vi "Kernel.vi"(0 "ref in":refnum<class "G#RemoteProxy.lvclass">, 1 "object name":string, 2 "option 1":bool, 3 "option 2":bool, 4 "depth":i32, 5 "error in (no error)":errorcluster, 6 "state":T3, 7 "option 3":bool, 8 "attributes in":variant[](array[variant]), 10 "class attributes in":variant[](array[variant])) -> (11 "class attributes out":variant[](array[variant]), 12 "class hierarchy":T1[](array[typedef]), 13 "attributes out":variant[](array[variant]), 14 "ref out":refnum<class "G#RemoteProxy.lvclass">, 15 "AttributeRefs":u32[](array[numeric]), 16 "static attribute ref":u32, 17 "output 1":bool, 18 "output 2":bool, 19 "error out":errorcluster)   [LabVIEW 2017, in "G#RemoteProxy.lvclass"]
doc: "Class kernel, creates and destroys the data value references of the class."
uses:
  G#RemoteProxy.lvclass
  G#Object/utils/G#Object_State.ctl
  G#Object/utils/G#Object_ClassHierarchy.ctl
  protected/ClassAttributesProxy.ctl
  G#Object/G#Object.lvclass
  ClassAttributesRef.ctl
  ObjectAttributesRef.ctl
  protected/ObjectAttributesProxy.ctl
  G#RemoteProxy.lvclass/G#RemoteProxy.ctl
  G#Object/utils/G#Object_ObjectInfoType.ctl
  G#Object/utils/G#Object_CreateMethod.ctl
  G#DebugServer/utils/TCPCommand.ctl
  G#DebugServer/G#DebugServer.lvclass
panel:
  in  "class attributes type":T2
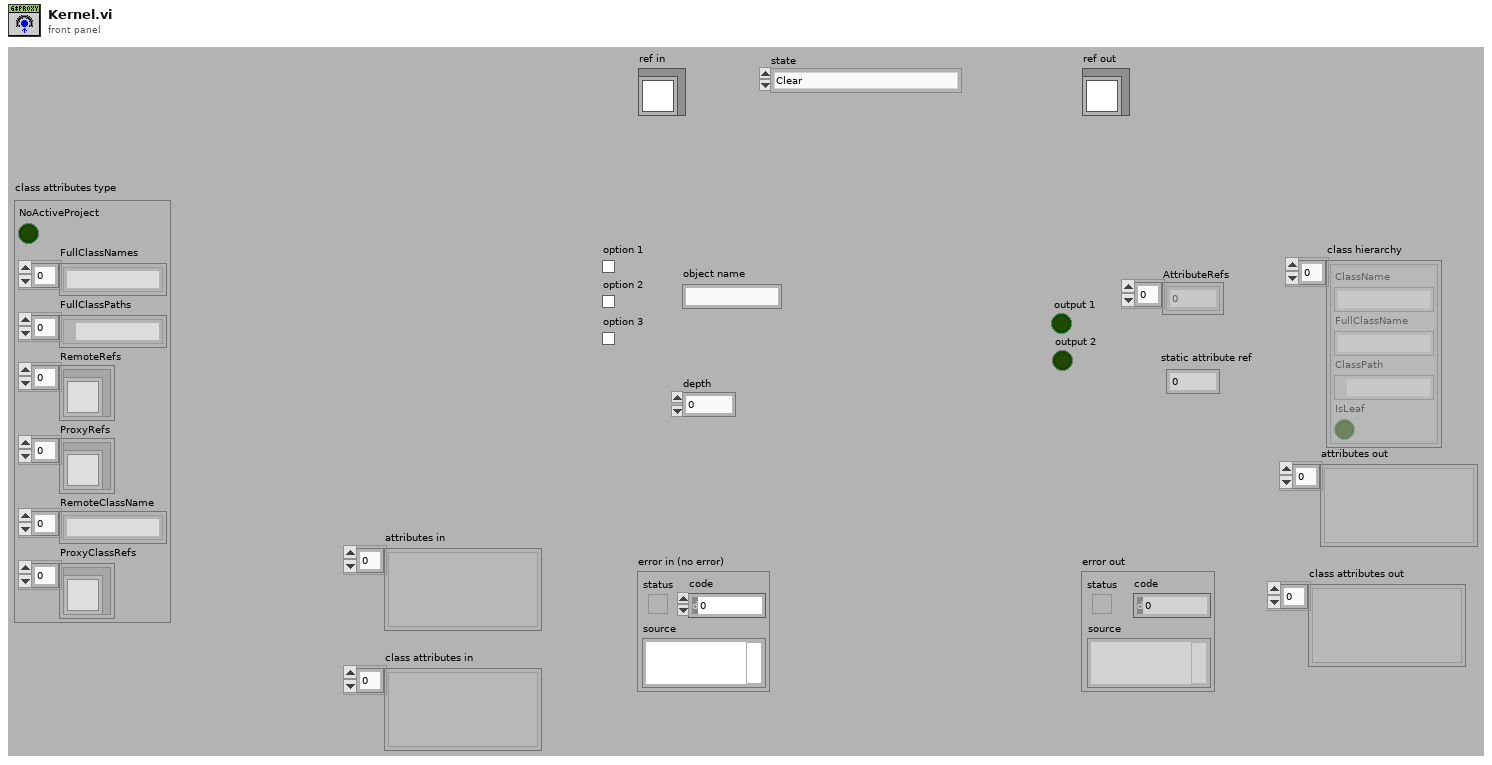
[diagram p1: front panel]
types:
  T1 = typedef "G#Object.lvclass/G#Object_ClassHierarchy.ctl" = cluster{"ClassName":string, "FullClassName":string, "ClassPath":path, "IsLeaf":bool}
  T2 = typedef "G#RemoteProxy.lvclass/ClassAttributesProxy.ctl" = cluster{"NoActiveProject":bool, "FullClassNames":string[], "FullClassPaths":path[], "RemoteRefs":refnum<class "G#Object.lvclass">[], "ProxyRefs":refnum<class "G#RemoteProxy.lvclass">[], "RemoteClassName":string[], "ProxyClassRefs":refnum<class "G#RemoteProxy.lvclass">[]}
  T3 = typedef "G#Object.lvclass/G#Object_State.ctl" = enum16{"Clear", "Create", "Delete", "Get class attributes", "Class hierarchy", "Get attribute value", "Set attribute value"}
  T4 = typedef "G#RemoteProxy.lvclass/ObjectAttributesRef.ctl" = refnum<data-value>
  T5 = typedef "G#RemoteProxy.lvclass/ClassAttributesRef.ctl" = refnum<data-value>
  T6 = typedef "G#RemoteProxy.lvclass/ObjectAttributesProxy.ctl" = cluster{"class hierarchy":T1[], "class name":string, "lvlib hierarchy":string[], "full class name":string, "id":u32, "owner":string, "RemoteRef":refnum<class "G#Object.lvclass">, "object name":string, "attributes":variant[], "connection ID":refnum<k5>, "address":u32, "occurrence":refnum<k4>, "ProxyClassRef":refnum<class "G#RemoteProxy.lvclass">, "InMemory?":bool, "ToString":string}
  T7 = typedef "G#Object.lvclass/G#Object_ObjectInfoType.ctl" = cluster{"ObjectName":string, "ObjectID":u32, "Users":i32, "Counter":bool, "AttributeRefs":u32[], "FullClassName":string, "ClassName":string, "CreateMethod":T8, "GenericDestructorExists":bool, "Owner":string}
  T8 = typedef "G#Object.lvclass/G#Object_CreateMethod.ctl" = enum16{"Create", "Create or look up existing", "Look up existing"}
  T9 = typedef "G#DebugServer.lvclass/TCPCommand.ctl" = u8
  T10 = cluster{"InMemory?":bool, "RemoteRef":refnum<class "G#Object.lvclass">}
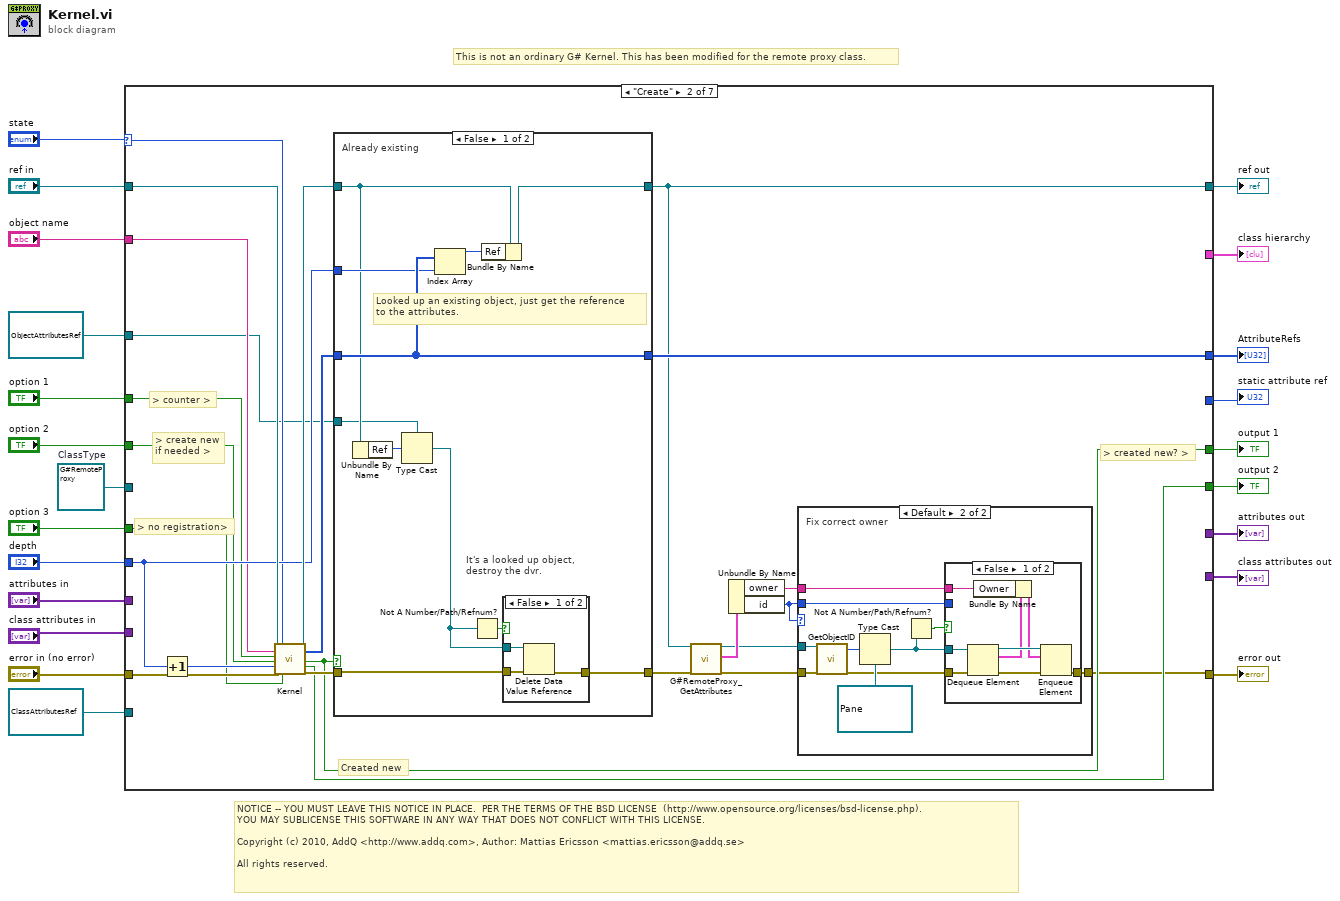
[diagram p0: block diagram]
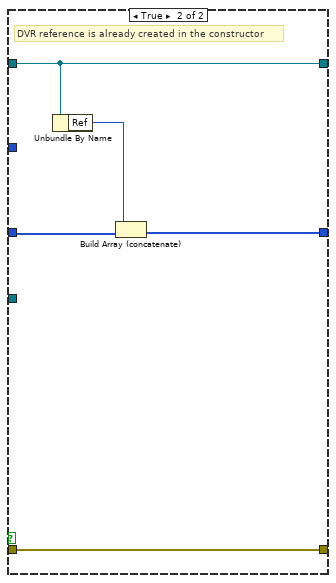
[diagram p6: hidden frame]
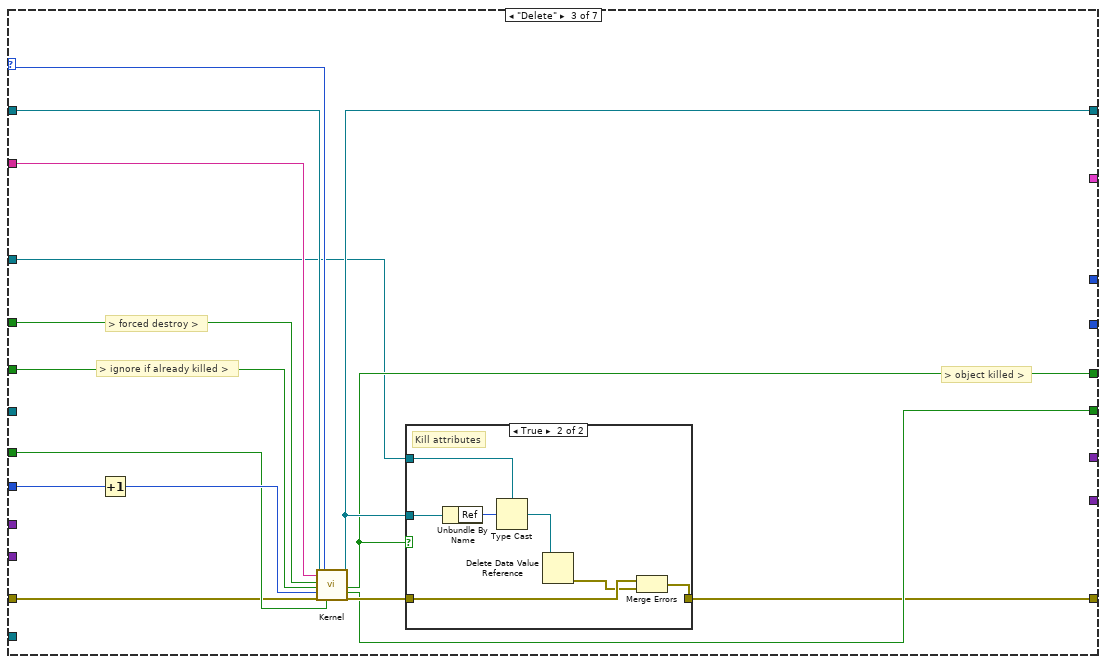
[diagram p7: hidden frame]
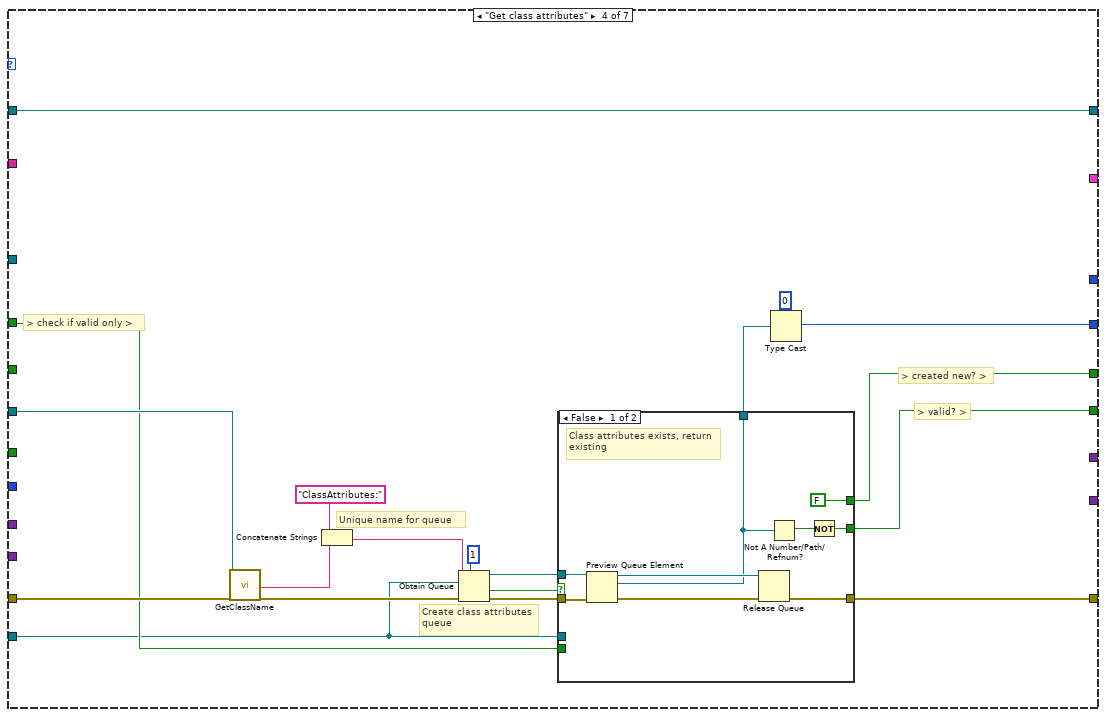
[diagram p9: hidden frame]
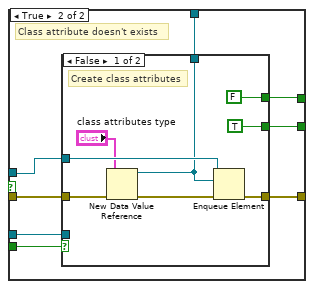
[diagram p10: hidden frame]
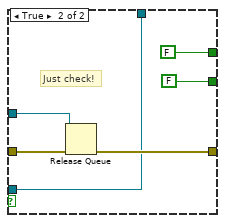
[diagram p11: hidden frame]
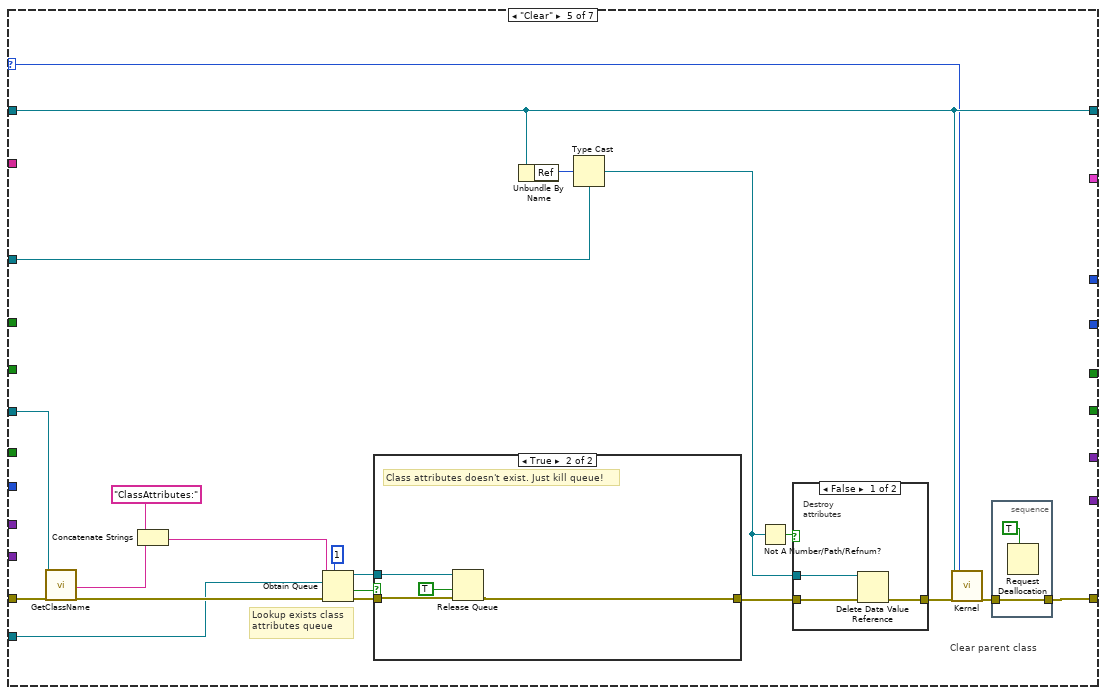
[diagram p12: hidden frame]
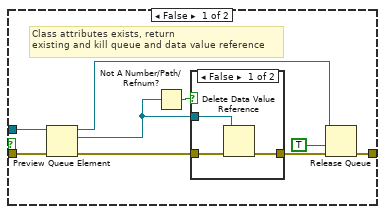
[diagram p14: hidden frame]
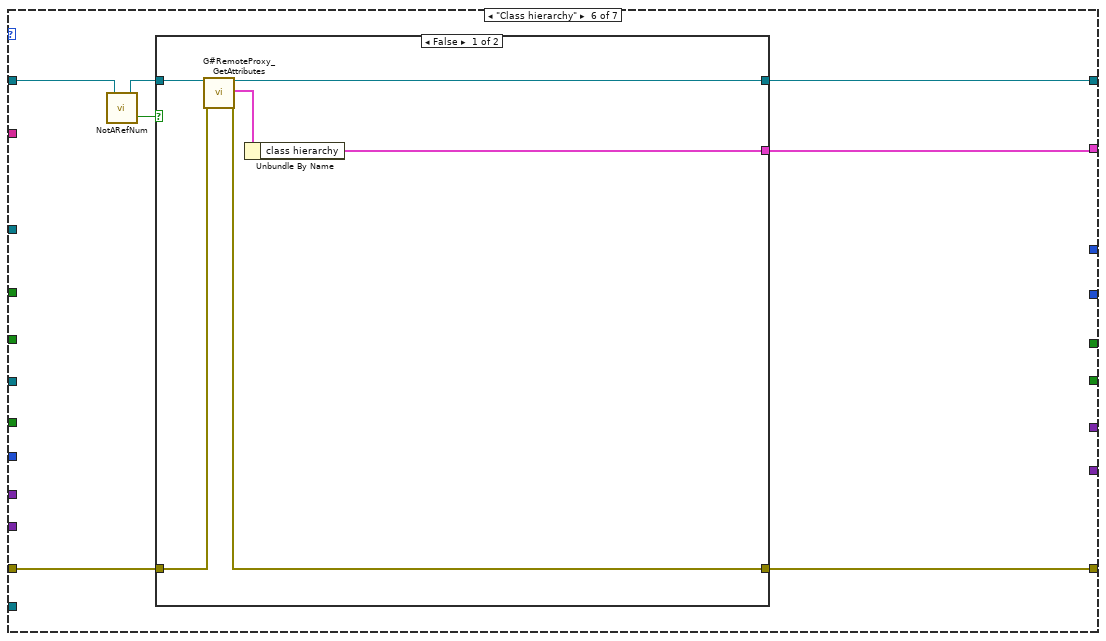
[diagram p16: hidden frame]
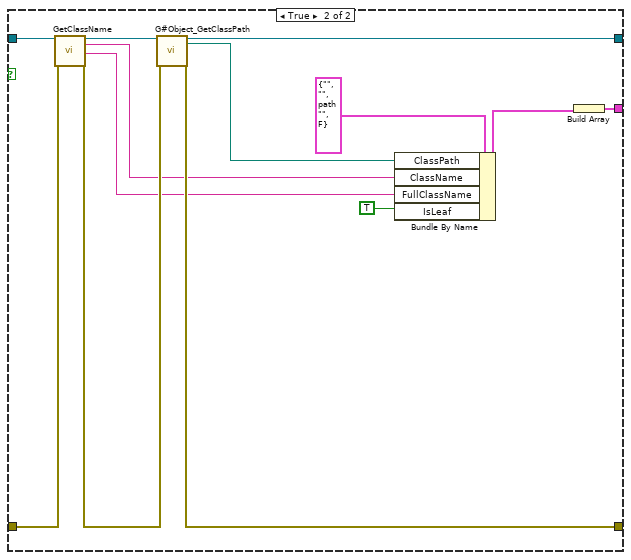
[diagram p17: hidden frame]
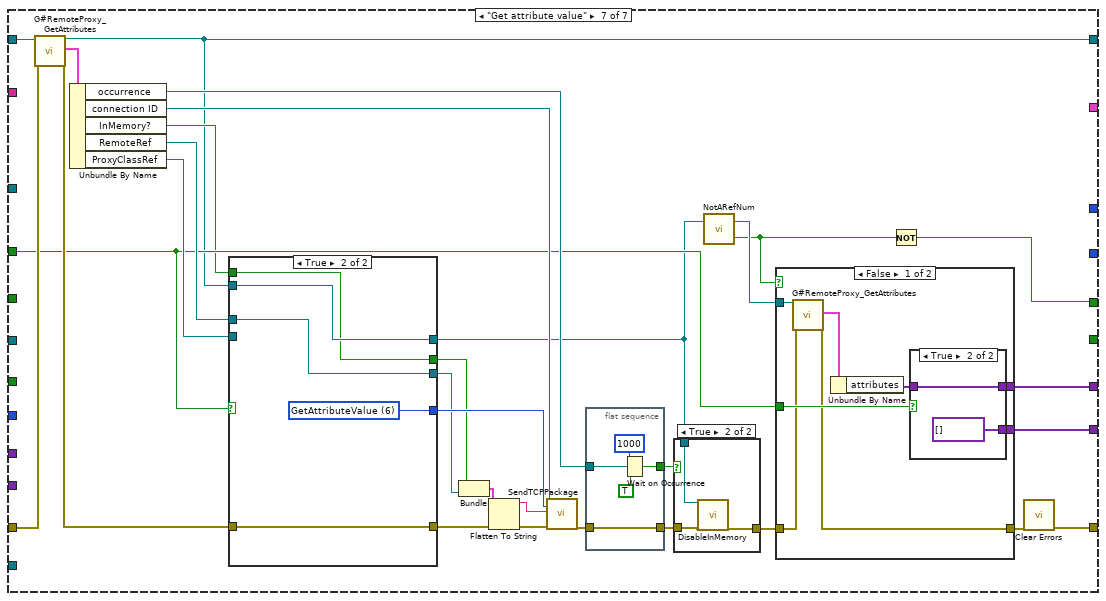
[diagram p18: hidden frame]
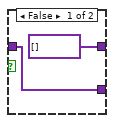
[diagram p19: hidden frame]
diagram:
  w11 = refnum<class "G#RemoteProxy.lvclass"> refnum  # ClassType
  # "This is not an ordinary G# Kernel. This has been modified for the remote proxy class."
  # "NOTICE -- YOU MUST LEAVE THIS NOTICE IN PLACE.  PER THE TERMS OF THE BSD LICENSE  (http://www.opensource.org/licenses/bsd-license.php).\nYOU MAY SUBLICENSE THIS SOFTWARE IN ANY WAY THAT DOES NOT CONFLICT WITH THIS LICENSE.\n\nCopyright (c) 2010, AddQ <http://www.addq.com>, Author: Mattias Ericsson <mattias.ericsson@addq.se>\n\nAll rights reserved."
  n1 = case shown="\"Create\"" "state" {
    selector: "state" -> [_ w41 w99 _ w169 _ _]
    tunnel: "ref in" -> [w24 w45 w96 w130 w170 w208 w261]
    tunnel: [w24 w31 w102 w130 w170 w212 w236] -> w20
    tunnel: "error in (no error)" -> [w23 w44 w91 w129 w182 w211 w260]
    tunnel: [w23 w33 w90 w119 w165 w210 w245] -> w18
    tunnel: "depth" -> [_ w43 w94 _ _ _ _]
    tunnel: "object name" -> [_ w42 w92 _ _ _ _]
    tunnel: "option 1" -> [_ w40 w100 w115 _ _ w246]
    tunnel: [_ w39 _ _ _ _ _] -> w14
    tunnel: [_ w37 w101 w112 _ _ w240] -> w13
    tunnel: [_ _ _ w120 _ _ _] -> w12
    tunnel: w11 -> [_ _ _ w117 w173 _ _]
    tunnel: T5 refnum ("data value reference") -> [_ _ _ w114 w172 _ _]
    tunnel: [_ _ _ _ _ w209 _] -> w9
    tunnel: [_ _ _ _ _ _ w247] -> w8
    tunnel: [_ _ _ _ _ _ w253] -> w7
    tunnel: "option 2" -> [_ w36 w98 _ _ _ _]
    tunnel: "option 3" -> [_ w34 w93 _ _ _ _]
    tunnel: [_ w35 w97 w113 _ _ _] -> w4
    tunnel: "attributes in" -> [_ _ _ _ _ _ _]
    tunnel: "class attributes in" -> [_ _ _ _ _ _ _]
    tunnel: T4 refnum ("attributes ref") -> [_ w25 w89 _ w163 _ _]
    frame Default {
    }
    frame "Create" {
      # "Created new"
      # "> no registration>"
      # "> create new\nif needed >"
      # "> created new? >"
      # "> counter >"
      n2 = Increment(x=w43) -> (x+1=w38:i32)
      n3 = call-parent "Kernel.vi"("reference in"=w45, "object name"=w42, "option 1"=w40, "option 2"=w36, "depth"=w38, "error in (no error)"=w44, "state"=w41, "option 3"=w34) -> ("reference out"=w46:refnum<class "G#RemoteProxy.lvclass">, "attribute refs"=w47:u32[], "output 1"=w37:bool, "output 2"=w35:bool, "error out"=w48:errorcluster)  [unwired: 3 in, 4 out]
      n4 = case shown="False" w37 {
        tunnel: w48 -> [w71 w84]
        tunnel: [w72 w84] -> w32
        tunnel: w46 -> [w75 w86]
        tunnel: [w79 w86] -> w31
        tunnel: w47 -> [w78 w88]
        tunnel: [w78 w87] -> w39
        tunnel: w43 -> [w77 _]
        tunnel: w25 -> [w73 _]
        frame False {
          # "It's a looked up object,\ndestroy the dvr."
          # "Looked up an existing object, just get the reference\nto the attributes."
          # "Already existing"
          n5 = Unbundle By Name(w75) -> ("Ref"=w74:u32)
          n6 = Type Cast(type=w73, x=w74) -> (*(type *) &x=w70:T4)
          n7 = Index Array(array=w78, index=w77) -> (element=w76:u32)
          n8 = Not A Number/Path/Refnum?(number/path/refnum=w70) -> (NaN/Path/Refnum?=w69:bool)
          n9 = Bundle By Name(cluster=w75, "Ref"=w76) -> (w79:refnum<class "G#RemoteProxy.lvclass">)
          n10 = case shown="False" w69 {
            tunnel: [w82 w83] -> w72
            tunnel: w71 -> [w81 w83]
            tunnel: w70 -> [w80 _]
            frame False {
              n11 = Delete Data Value Reference(data value reference=w80, error in=w81) -> (error out=w82:errorcluster)  [unwired: 1 out]
            }
            frame True {
            }
          }
        }
        frame True {
          # "DVR reference is already created in the constructor"
          n12 = Unbundle By Name(w86) -> ("Ref"=w85:u32)
          n13 = Build Array (concatenate)(w85, w88) -> (w87:u32[])
        }
      }
      n14 = call "G#RemoteProxy_GetAttributes.vi"("reference in"=w31, "error in (no error)"=w32) -> ("reference out"=w27:refnum<class "G#RemoteProxy.lvclass">, "attributes"=w28:T6, "error out"=w30:errorcluster)  [unwired: 14 in, 1 out]
      n15 = Unbundle By Name(w28) -> ("owner"=w29:string, "id"=w26:u32)
      n16 = case shown="Default" w26 {
        tunnel: [w49 w56] -> w33
        tunnel: w30 -> [w49 w55]
        tunnel: w29 -> [_ w52]
        tunnel: w26 -> [_ w53]
        tunnel: w27 -> [_ w54]
        frame 0 {
          # "Class attribute object,\ndon't do anything"
        }
        frame Default {
          # "Fix correct owner"
          n17 = call-dynamic "GetObjectID.vi"("reference in"=w54, "error in (no error)"=w55) -> ("object ID"=w58:u32, "error out"=w57:errorcluster)  [unwired: 15 in, 1 out]
          n18 = Type Cast(type=refnum<queue> refnum ("queue out"), x=w58) -> (*(type *) &x=w51:refnum<queue>)
          n19 = Not A Number/Path/Refnum?(number/path/refnum=w51) -> (NaN/Path/Refnum?=w50:bool)
          n20 = case shown="False" w50 {
            tunnel: w57 -> [w67 w68]
            tunnel: [w64 w68] -> w56
            tunnel: w53 -> [_ _]
            tunnel: w52 -> [w61 _]
            tunnel: w51 -> [w60 _]
            frame False {
              n21 = Dequeue Element(queue=w60, error in (no error)=w67) -> (queue out=w65:refnum<queue>, element=w63:T7, error out=w66:errorcluster)  [unwired: 1 in, 1 out]
              n22 = Bundle By Name(cluster=w63, "Owner"=w61) -> (w62:T7)
              n23 = Enqueue Element(queue=w65, element=w62, error in (no error)=w66) -> (error out=w64:errorcluster)  [unwired: 1 in, 2 out]
            }
            frame True {
            }
          }
        }
      }
    }
    frame "Delete" {
      # "> ignore if already killed >"
      # "> object killed >"
      # "> forced destroy >"
      n24 = Increment(x=w94) -> (x+1=w95:i32)
      n25 = call-parent "Kernel.vi"("reference in"=w96, "object name"=w92, "option 1"=w100, "option 2"=w98, "depth"=w95, "error in (no error)"=w91, "state"=w99, "option 3"=w93) -> ("reference out"=w102:refnum<class "G#RemoteProxy.lvclass">, "output 1"=w101:bool, "output 2"=w97:bool, "error out"=w103:errorcluster)  [unwired: 3 in, 5 out]
      n26 = case shown="True" w101 {
        tunnel: w103 -> [w104 w110]
        tunnel: w102 -> [_ w111]
        tunnel: [w104 w108] -> w90
        tunnel: w89 -> [_ w106]
        frame False {
        }
        frame True {
          # "Kill attributes"
          n27 = Unbundle By Name(w111) -> ("Ref"=w107:u32)
          n28 = Type Cast(type=w106, x=w107) -> (*(type *) &x=w105:T4)
          n29 = Delete Data Value Reference(data value reference=w105) -> (error out=w109:errorcluster)  [unwired: 1 in, 1 out]
          n30 = Merge Errors(w110, w109) -> (w108:errorcluster)
        }
      }
    }
    frame "Get class attributes" {
      # "> valid? >"
      # "> created new? >"
      # "> check if valid only >"
      # "Unique name for queue"
      # "Create class attributes\nqueue"
      n31 = call-dynamic "GetClassName.vi"("reference in"=w117, "error in (no error)"=w129) -> ("full class name"=w118:string, "error out"=w124:errorcluster)  [unwired: 13 in, 3 out]
      n32 = Concatenate Strings("ClassAttributes:" ("string"), w118) -> (w123:string)
      n33 = Obtain Queue(max queue size (-1, unlimited)=1, name (unnamed)=w123, element data type=w114, error in (no error)=w124) -> (queue out=w125:refnum<queue>, created new?=w116:bool, error out=w126:errorcluster)  [unwired: 1 in]
      n34 = case shown="False" w116 {
        tunnel: w126 -> [w139 w147]
        tunnel: w125 -> [w138 w146]
        tunnel: [w137 w144] -> w119
        tunnel: [w133 w145] -> w121
        tunnel: w115 -> [_ w143]
        tunnel: w114 -> [_ w142]
        tunnel: [w132 w141] -> w113
        tunnel: [FALSE w140] -> w112
        frame False {
          # "Class attributes exists, return\nexisting"
          n35 = Preview Queue Element(queue=w138, error in (no error)=w139) -> (queue out=w135:refnum<queue>, element=w133:T5, error out=w136:errorcluster)  [unwired: 1 in, 1 out]
          n36 = Release Queue(queue=w135, error in (no error)=w136) -> (error out=w137:errorcluster)  [unwired: 1 in, 2 out]
          n37 = Not A Number/Path/Refnum?(number/path/refnum=w133) -> (NaN/Path/Refnum?=w131:bool)
          n38 = Not(x=w131) -> (.not. x?=w132:bool)
        }
        frame True {
          # "Class attribute doesn't exists"
          n39 = case shown="False" w143 {
            tunnel: w147 -> [w155 w161]
            tunnel: w146 -> [w153 w160]
            tunnel: [w152 w158] -> w145
            tunnel: [w151 w159] -> w144
            tunnel: w142 -> [_ w158]
            tunnel: [TRUE FALSE] -> w141
            tunnel: [FALSE FALSE] -> w140
            frame False {
              # "Create class attributes"
              n40 = New Data Value Reference(data value="class attributes type", error in=w155) -> (data value reference=w152:refnum<data-value>, error out=w154:errorcluster)
              n41 = Enqueue Element(queue=w153, element=w152, error in (no error)=w154) -> (error out=w151:errorcluster)  [unwired: 1 in, 2 out]
            }
            frame True {
              # "Just check!"
              n42 = Release Queue(queue=w160, error in (no error)=w161) -> (error out=w159:errorcluster)  [unwired: 1 in, 2 out]
            }
          }
        }
      }
      n43 = Type Cast(type=u32 0, x=w121) -> (*(type *) &x=w120:u32)
    }
    frame "Clear" {
      # "Clear parent class"
      # "Lookup exists class\nattributes queue"
      n44 = call-dynamic "GetClassName.vi"("reference in"=w173, "error in (no error)"=w182) -> ("full class name"=w174:string, "error out"=w176:errorcluster)  [unwired: 13 in, 3 out]
      n45 = Concatenate Strings("ClassAttributes:" ("string"), w174) -> (w175:string)
      n46 = Obtain Queue(max queue size (-1, unlimited)=1, name (unnamed)=w175, element data type=w172, error in (no error)=w176) -> (queue out=w177:refnum<queue>, created new?=w178:bool, error out=w179:errorcluster)  [unwired: 1 in]
      n47 = case shown="True" w178 {
        tunnel: w179 -> [w192 w204]
        tunnel: w177 -> [w193 w205]
        tunnel: [w195 w203] -> w168
        frame False {
          # "Class attributes exists, return\nexisting and kill queue and data value reference"
          n48 = Preview Queue Element(queue=w193, error in (no error)=w192) -> (queue out=w190:refnum<queue>, element=w189:T5, error out=w191:errorcluster)  [unwired: 1 in, 1 out]
          n49 = Not A Number/Path/Refnum?(number/path/refnum=w189) -> (NaN/Path/Refnum?=w196:bool)
          n50 = case shown="False" w196 {
            tunnel: w191 -> [w200 w201]
            tunnel: [w199 w201] -> w194
            tunnel: w189 -> [w198 _]
            frame False {
              n51 = Delete Data Value Reference(data value reference=w198, error in=w200) -> (error out=w199:errorcluster)  [unwired: 1 out]
            }
            frame True {
            }
          }
          n52 = Release Queue(queue=w190, force destroy? (F)=TRUE, error in (no error)=w194) -> (error out=w195:errorcluster)  [unwired: 2 out]
        }
        frame True {
          # "Class attributes doesn't exist. Just kill queue!"
          n53 = Release Queue(queue=w205, force destroy? (F)=TRUE, error in (no error)=w204) -> (error out=w203:errorcluster)  [unwired: 2 out]
        }
      }
      n54 = Unbundle By Name(w170) -> ("Ref"=w164:u32)
      n55 = Type Cast(type=w163, x=w164) -> (*(type *) &x=w162:T4)
      n56 = Not A Number/Path/Refnum?(number/path/refnum=w162) -> (NaN/Path/Refnum?=w171:bool)
      n57 = case shown="False" w171 {
        tunnel: w162 -> [w185 _]
        tunnel: w168 -> [w187 w188]
        tunnel: [w186 w188] -> w167
        frame False {
          # "Destroy\nattributes"
          n58 = Delete Data Value Reference(data value reference=w185, error in=w187) -> (error out=w186:errorcluster)  [unwired: 1 out]
        }
        frame True {
        }
      }
      n59 = call-parent "Kernel.vi"("reference in"=w170, "error in (no error)"=w167, "state"=w169) -> ("error out"=w166:errorcluster)  [unwired: 8 in, 8 out]
      n60 = stacked-sequence {
        tunnel: w166 -> [w183]
        tunnel: [w183] -> w165
        frame #0 {
          n61 = Request Deallocation(TRUE ("flag")) -> ()
        }
      }
    }
    frame "Class hierarchy" {
      n62 = call-dynamic "NotARefNum.vi"("reference in"=w208) -> ("not a refnum?"=w206:bool, "reference out"=w207:refnum<class "G#RemoteProxy.lvclass">)  [unwired: 1 in]
      n63 = case shown="False" w206 {
        tunnel: [w218 w231] -> w212
        tunnel: w211 -> [w217 w223]
        tunnel: [w216 w230] -> w210
        tunnel: [w214 w229] -> w209
        tunnel: w207 -> [w213 w225]
        frame False {
          n64 = call "G#RemoteProxy_GetAttributes.vi"("reference in"=w213, "error in (no error)"=w217) -> ("reference out"=w218:refnum<class "G#RemoteProxy.lvclass">, "attributes"=w215:T6, "error out"=w216:errorcluster)  [unwired: 14 in, 1 out]
          n65 = Unbundle By Name(w215) -> ("class hierarchy"=w214:T1[])
        }
        frame True {
          n66 = call-dynamic "GetClassName.vi"("reference in"=w225, "error in (no error)"=w223) -> ("reference out"=w224:refnum<class "G#RemoteProxy.lvclass">, "class name"=w220:string, "full class name"=w219:string, "error out"=w222:errorcluster)  [unwired: 13 in, 1 out]
          n67 = call-dynamic "G#Object_GetClassPath.vi"("reference in"=w224, "error in (no error)"=w222) -> ("reference out"=w231:refnum<class "G#RemoteProxy.lvclass">, "class path"=w226:path, "error out"=w230:errorcluster)  [unwired: 15 in]
          n68 = Bundle By Name(cluster=T1 {"ClassName"="", "FullClassName"="", "ClassPath"=path "", "IsLeaf"=FALSE} ("ClassHierarchy"), "ClassPath"=w226, "ClassName"=w220, "FullClassName"=w219, "IsLeaf"=TRUE) -> (w227:T1)
          n69 = Build Array(w227) -> (w229:T1[])
        }
      }
    }
    frame "Get attribute value" {
      n70 = call "G#RemoteProxy_GetAttributes.vi"("reference in"=w261, "error in (no error)"=w260) -> ("reference out"=w236:refnum<class "G#RemoteProxy.lvclass">, "attributes"=w259:T6, "error out"=w252:errorcluster)  [unwired: 14 in, 1 out]
      n71 = Unbundle By Name(w259) -> ("occurrence"=w254:refnum<k4>, "connection ID"=w256:refnum<k5>, "InMemory?"=w241:bool, "RemoteRef"=w250:refnum<class "G#Object.lvclass">, "ProxyClassRef"=w248:refnum<class "G#RemoteProxy.lvclass">)
      n72 = case shown="True" w246 {
        tunnel: w252 -> [w285 w291]
        tunnel: [w284 w291] -> w251
        tunnel: w250 -> [_ w290]
        tunnel: [w282 w290] -> w243
        tunnel: [w281 w289] -> w249
        tunnel: w248 -> [w286 _]
        tunnel: w236 -> [_ w288]
        tunnel: [w280 w288] -> w233
        tunnel: [w279 w287] -> w244
        tunnel: w241 -> [_ w287]
        frame False {
          w281 = T9 8 items=["GarbageCollect", "GetAllObjects", "GetAllObjectsReply", "CleanUp", "G#Event", "RegisterClient", "GetAttributeValue", "GetAttributeValueReply", "GetClassAttributeValue", "GetClassAttributeValueReply", "GetToStringValue", "GetToStringValueReply", "GetClassHierarchy", "GetClassHierarchyReply"] ("Command")
          n73 = call "G#RemoteProxy_GetAttributes.vi"("reference in"=w286, "error in (no error)"=w285) -> ("reference out"=w280:refnum<class "G#RemoteProxy.lvclass">, "attributes"=w283:T6, "error out"=w284:errorcluster)  [unwired: 14 in, 1 out]
          n74 = Unbundle By Name(w283) -> ("InMemory?"=w279:bool, "RemoteRef"=w282:refnum<class "G#Object.lvclass">)
        }
        frame True {
          w289 = T9 6 items=["GarbageCollect", "GetAllObjects", "GetAllObjectsReply", "CleanUp", "G#Event", "RegisterClient", "GetAttributeValue", "GetAttributeValueReply", "GetClassAttributeValue", "GetClassAttributeValueReply", "GetToStringValue", "GetToStringValueReply", "GetClassHierarchy", "GetClassHierarchyReply"] ("Command")
        }
      }
      n75 = Bundle("InMemory?"=w244, "RemoteRef"=w243) -> (w242:T10)  [unwired: 1 in]
      n76 = Flatten To String(anything=w242, error in (no error)=w251) -> (data string=w257:string, error out=w258:errorcluster)  [unwired: 2 in, 1 out]
      n77 = call "SendTCPPackage.vi"("connection ID"=w256, "command"=w249, "data"=w257, "error in (no error)"=w258) -> ("error out"=w255:errorcluster)  [unwired: 15 in]
      n78 = flat-sequence {
        tunnel: w255 -> [w294]
        tunnel: w254 -> [w296]
        tunnel: [w294] -> w238
        tunnel: [w293] -> w239
        frame #0 {
          n79 = Wait on Occurrence(1:TRUE ("ignore previous (T)"), 2:w296, 3:1000 ("ms timeout (-1)")) -> (0:w293:bool)
        }
      }
      n80 = case shown="True" w239 {
        tunnel: w238 -> [w275 w278]
        tunnel: [w275 w277] -> w237
        tunnel: w233 -> [_ w276]
        frame False {
        }
        frame True {
          n81 = call "DisableInMemory.vi"("reference in"=w276, "error in (no error)"=w278) -> ("error out"=w277:errorcluster)  [unwired: 16 in, 1 out]
        }
      }
      n82 = call-dynamic "NotARefNum.vi"("reference in"=w233) -> ("not a refnum?"=w232:bool, "reference out"=w234:refnum<class "G#RemoteProxy.lvclass">)  [unwired: 1 in]
      n83 = case shown="False" w232 {
        tunnel: [w268 _] -> w253
        tunnel: [w267 _] -> w247
        tunnel: w246 -> [w265 _]
        tunnel: w237 -> [w264 w274]
        tunnel: [w263 w274] -> w235
        tunnel: w234 -> [w262 _]
        frame False {
          n84 = call "G#RemoteProxy_GetAttributes.vi"("reference in"=w262, "error in (no error)"=w264) -> ("attributes"=w269:T6, "error out"=w263:errorcluster)  [unwired: 14 in, 2 out]
          n85 = Unbundle By Name(w269) -> ("attributes"=w266:variant[])
          n86 = case shown="True" w265 {
            tunnel: [w271 variant[] [] ("class attributes")] -> w268
            tunnel: w266 -> [w271 w272]
            tunnel: [variant[] [] ("attributes") w272] -> w267
            frame False {
            }
            frame True {
            }
          }
        }
        frame True {
        }
      }
      n87 = Not(x=w232) -> (.not. x?=w240:bool)
      n88 = call <vilib>:"Clear Errors.vi"("error in (no error)"=w235) -> ("error out"=w245:errorcluster)  [unwired: 5 in, 1 out]
    }
  }
  "error out" <- w18
  "ref out" <- w20
  "AttributeRefs" <- w14
  "static attribute ref" <- w12
  "output 1" <- w13
  "output 2" <- w4
  "class hierarchy" <- w9
  "attributes out" <- w8
  "class attributes out" <- w7
